vi "Test At Least Two Calls Any Inputs Pass.vi"(8 "error in (no error)":errorcluster, 11 "Test Case In":refnum<class "Expectation Message Test.lvclass">) -> (0 "error out":errorcluster, 3 "Test Case Out":refnum<class "Expectation Message Test.lvclass">)   [LabVIEW 2020, in "Expectation Message Test.lvclass"]
uses:
  Expectation Message Test.lvclass
  C:/Program Files (x86)/National Instruments/LabVIEW 2020/vi.lib/Astemes/LUnit/Test Case.lvclass
  Test Doubles/Test Interface Responsive Mock/Test Interface Mock.lvclass
  C:/git/astemes-lmock/source/Framework/Mock/LMock Mock.lvclass
  source/Expectations/At Least/At Least Ignore Inputs.vi
  C:/git/astemes-lmock/tests/Test Doubles/Test Interface Responsive Mock/Test Interface Mock.lvclass
  C:/git/astemes-lmock/tests/Test Doubles/Test Interface/Test Interface.lvclass
  Expectation Test/Expectation Test.lvclass
  source/Framework/LMock API.lvlib
  source/Expectations/At Least/At Least.lvlib
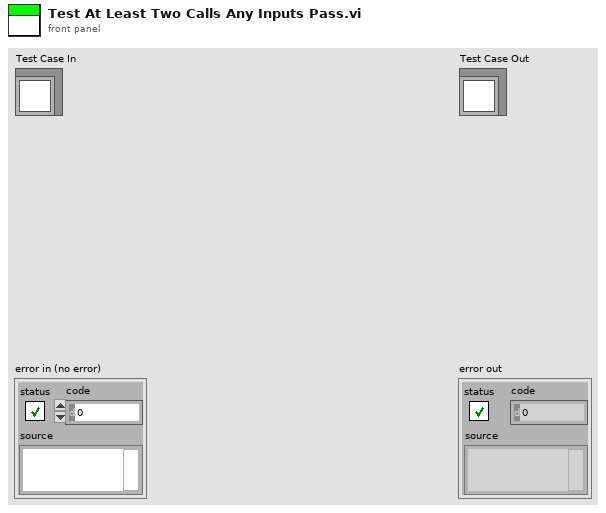
[diagram p1: front panel]
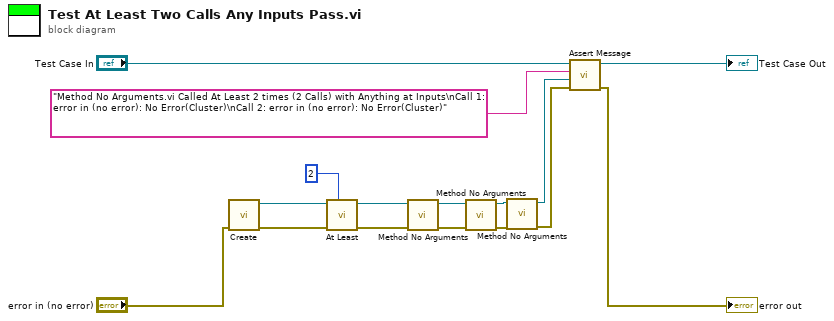
[diagram p0: block diagram]
diagram:
  n1 = call "Create.vi"("error in (no error)"="error in (no error)") -> ("error out"=w13:errorcluster, "Test Interface Mock Out"=w11:refnum<class "Test Interface Mock.lvclass">)  [unwired: 9 in]
  n2 = call-poly "At Least.vi"("Minimum Number of Calls"=u32 2 ("Expected Number of Calls"), "error in (no error)"=w13, "Mock in"=w11) -> ("error out"=w12:errorcluster, "Mock out"=w10:refnum<class "Test Interface Mock.lvclass">)  [unwired: 7 in]
  n3 = call-dynamic "Method No Arguments.vi"("error in (no error)"=w12, "Mock In"=w10) -> ("error out"=w9:errorcluster, "Mock Out"=w5:refnum<class "Test Interface Mock.lvclass">)  [unwired: 8 in]
  n4 = call-dynamic "Method No Arguments.vi"("error in (no error)"=w9, "Mock In"=w5) -> ("error out"=w6:errorcluster, "Mock Out"=w2:refnum<class "Test Interface Mock.lvclass">)  [unwired: 8 in]
  n5 = call-dynamic "Method No Arguments.vi"("error in (no error)"=w6, "Mock In"=w2) -> ("error out"=w3:errorcluster, "Mock Out"=w1:refnum<class "Test Interface Mock.lvclass">)  [unwired: 8 in]
  n6 = call "Assert Message.vi"("error in (no error)"=w3, "Mock"=w1, "Message"="Method No Arguments.vi Called At Least 2 times (2 Calls) with Anything at Inputs\nCall 1: error in (no error): No Error(Cluster)\nCall 2: error in (no error): No Error(Cluster)", "LUnit Test Case In"="Test Case In") -> ("error out"=→"error out":errorcluster, "LUnit Test Case Out"=→"Test Case Out":refnum<class "Expectation Message Test.lvclass">)  [unwired: 6 in]
